vi "OAT Online Spectral Map with Resample.vi"(0 "scaled signal [EU]":waveform(dbl)={"t0"=timestamp(0 s since 1904-01-01), "dt"=0.0, "Y"=[]}, 1 "dB On (T)":bool=TRUE, 2 "reset? (True)":bool=TRUE, 5 "speed profile":T5 {"speed [RPM]" format="%.2f"; "time [s]" format="%.2f"}, 7 "pulse/revolution (1)":i32=1, 11 "error in (no error)":errorcluster, 12 "max order":i32, 13 "config":T1 {"range (auto)"."step" format="%.2f"; "range (auto)"."end" format="%.2f"; "range (auto)"."start" format="%.2f"}, 14 "window info":T2={"window type"=10, "window length"=2048} {"window type" items=["None"=0, "Hanning"=1, "Hamming"=2, "Blackman-Harris"=3, "Exact Blackman"=4, "Blackman"=5, "Flat Top"=6, "4 Term B-Harris"=7, "7 Term B-Harris"=8, "Low Sidelobe"=9, "Gaussian"=62]; "window length" min=0}) -> (4 "spectral map":dbl[][](array[numeric]) format="%.2f", 6 "scales":T4 {"Y scale"."multiplier" format="%.2f"; "Y scale"."offset" format="%.2f"; "X scale"."multiplier" format="%.2f"; "X scale"."offset" format="%.2f"}, 8 "unit labels":T3, 10 "finished":bool, 15 "error out":errorcluster)   [LabVIEW 2017]
doc: "Computes the <B>spectral map</B> of <B>scaled signal [EU]</B> based on the resampling method. This VI continuously computes <B>spectral map</B>."
uses:
  <vilib>/addons/Sound and Vibration/Order Analysis/Tach Process/SubVIs/speed profile.ctl
  <vilib>/addons/Sound and Vibration/Order Analysis/Ref Gabor Order Tracking/window information.ctl
  <vilib>/addons/Sound and Vibration/Order Analysis/Resample Order Tracking/OAT Convert to Even Angle Signal (1 Channel).vi
  <vilib>/Waveform/WDTOps.llb/WDT Waveform Duration DBL.vi
  <vilib>/addons/Sound and Vibration/Order Analysis/Resample Order Tracking/SoundVib_Resampling.lvlib
  <vilib>/addons/Sound and Vibration/Order Analysis/Resample Order Tracking/SoundVib_OrderTracking.lvlib
  <vilib>/addons/Sound and Vibration/Order Analysis/Gabor Order Tracking/SoundVib_Gabor.lvlib
  <vilib>/addons/Sound and Vibration/Order Analysis/Tach Process/SoundVib_TachProcess.lvlib
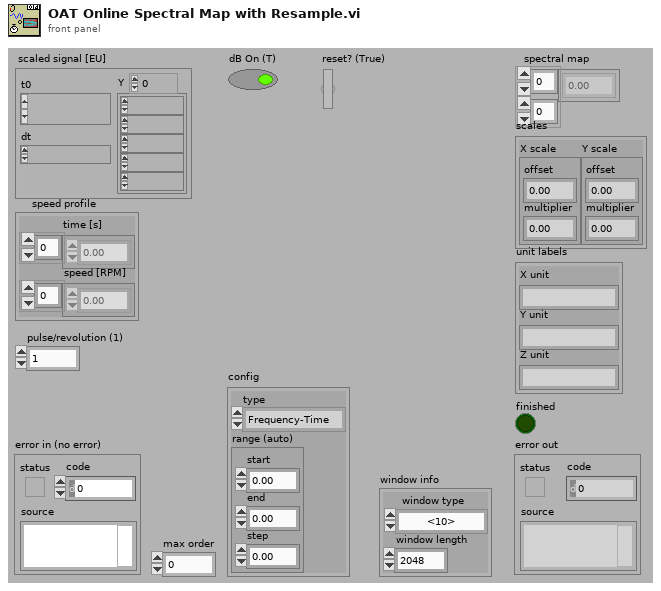
[diagram p1: front panel]
types:
  T1 = cluster{"type":enum16{"Frequency-Time", "Frequency-RPM", "Order-RPM"}, "range (auto)":cluster{"start":dbl, "end":dbl, "step":dbl}}
  T2 = typedef "SoundVib_Gabor.lvlib/window information.ctl" = cluster{"window type":u32, "window length":i32}
  T3 = cluster{"X unit":string, "Y unit":string, "Z unit":string}
  T4 = cluster{"X scale":cluster{"offset":dbl, "multiplier":dbl}, "Y scale":cluster{"offset":dbl, "multiplier":dbl}}
  T5 = typedef "SoundVib_TachProcess.lvlib/speed profile.ctl" = cluster{"time [s]":dbl[], "speed [RPM]":dbl[]}
  T6 = cluster{"Z axis unit label":string, "Z axis unit label":string, "Z axis unit label":string}
  T7 = cluster{"type":enum16{"Frequency-Time", "Frequency-RPM", "Order-RPM"}, "range":cluster{"start":dbl, "end":dbl, "step":dbl}}
  T8 = enum16{"Frequency-Time", "Frequency-RPM", "Order-RPM"}
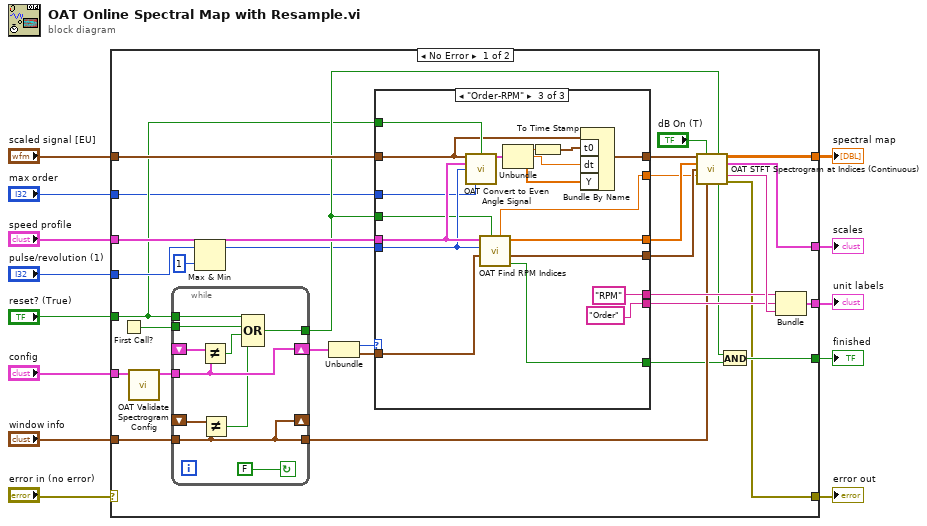
[diagram p0: block diagram]
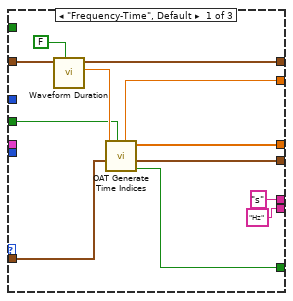
[diagram p2: hidden frame]
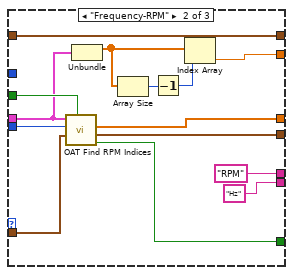
[diagram p3: hidden frame]
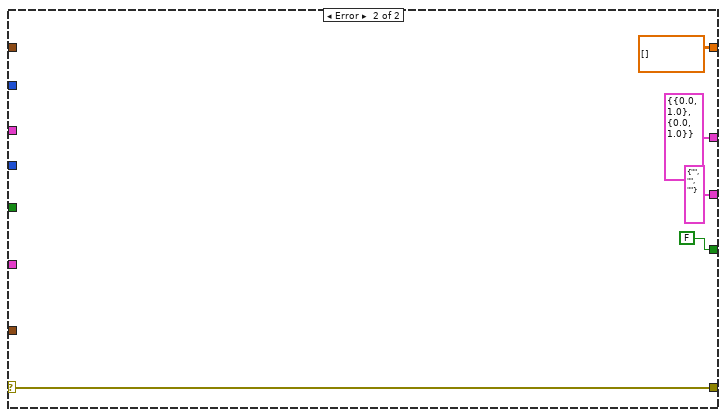
[diagram p4: hidden frame]
diagram:
  n1 = case shown="No Error" "error in (no error)" {
    selector: "error in (no error)" -> [_ w104]
    tunnel: "speed profile" -> [w44 _]
    tunnel: "scaled signal [EU]" -> [w43 _]
    tunnel: "pulse/revolution (1)" -> [w42 _]
    tunnel: [w36 dbl[][] [] ("spectral map")] -> w10
    tunnel: "window info" -> [w31 _]
    tunnel: [w27 FALSE] -> w8
    tunnel: [w26 T6 {"Z axis unit label"="", "Z axis unit label"="", "Z axis unit label"=""}] -> w7
    tunnel: "config" -> [w25 _]
    tunnel: "reset? (True)" -> [w23 _]
    tunnel: [w19 T4 {"X scale"={"offset"=0.0, "multiplier"=1.0}, "Y scale"={"offset"=0.0, "multiplier"=1.0}} ("scales")] -> w4
    tunnel: "max order" -> [w17 _]
    tunnel: [w16 w104] -> w1
    frame No Error {
      n2 = First Call?() -> (First Call?: T/F=w22:bool)
      n3 = call <vilib>:"OAT Validate Spectrogram Config.vi"("config"=w25) -> ("config"=w24:T7)  [unwired: 10 in]
      n4 = while {
        tunnel: w24 -> [w49]
        tunnel: w22 -> [w54]
        tunnel: w23 -> [w53]
        tunnel: [w51] -> w39
        shift-right: [w49] -> w37
        shift-left: _ -> [w48]
        shift-right: [w47] -> _
        shift-left: _ -> [w46]
        tunnel: w31 -> [w47]
        tunnel: [w47] -> w30
        stop <- FALSE continue-if-true
        n5 = Not Equal?(x=w48, y=w49) -> (x != y?=w52:bool)
        n6 = Not Equal?(x=w46, y=w47) -> (x != y?=w45:bool)
        n7 = Compound Arithmetic op=OR(w53, w54, w52, w45) -> (w51:bool)
      }
      n8 = Max & Min(x=w42, y=1) -> (max(x,y)=w15:i32)  [unwired: 1 out]
      n9 = Unbundle(w37) -> ("type"=w41:T8, "range"=w38:cluster{"start":dbl, "end":dbl, "step":dbl})
      n10 = case shown="\"Order-RPM\"" w41 {
        tunnel: w43 -> [w63 w78 w88]
        tunnel: [w62 w78 w83] -> w40
        tunnel: w44 -> [_ w71 w99]
        tunnel: w38 -> [w64 w80 w98]
        tunnel: w15 -> [_ w79 w97]
        tunnel: [w58 w77 w96] -> w21
        tunnel: w39 -> [w56 w76 w95]
        tunnel: [w59 w75 w94] -> w28
        tunnel: [w57 w74 w93] -> w20
        tunnel: ["s" ("Z axis unit label") "RPM" ("Z axis unit label") "RPM" ("Z axis unit label")] -> w33
        tunnel: ["Hz" ("Z axis unit label") "Hz" ("Z axis unit label") "Order" ("Z axis unit label")] -> w32
        tunnel: w17 -> [_ _ w82]
        tunnel: w23 -> [_ _ w90]
        tunnel: [w55 w67 w89] -> w18
        frame "Frequency-Time", Default {
          n11 = call-poly <vilib>:"Waveform Duration.vi"("open interval? (T)"=FALSE, "waveform in"=w63) -> ("duration"=w60:dbl, "waveform out"=w62:waveform(dbl))  [unwired: 7 in, 1 out]
          n12 = call <vilib>:"OAT Generate Time Indices.vi"("reset? (True)"=w56, "steps"=w64, "duration"=w60) -> ("finished"=w59:bool, "scale"=w57:cluster{"offset":dbl, "multiplier":dbl}, "time indices"=w58:dbl[], "signal processed"=w55:dbl)  [unwired: 5 in]
        }
        frame "Frequency-RPM" {
          n13 = call <vilib>:"OAT Find RPM Indices.vi"("reset? (True)"=w76, "RPM range"=w80, "pulse/revolution (1)"=w79, "speed profile"=w71) -> ("finished"=w75:bool, "RPM scale"=w74:cluster{"offset":dbl, "multiplier":dbl}, "time indices"=w77:dbl[])  [unwired: 3 in, 2 out]
          n14 = Unbundle(w71) -> ("time [s]"=w70:dbl[])  [unwired: 1 out]
          n15 = Array Size(array=w70) -> (size(s)=w69:i32)
          n16 = Decrement(x=w69) -> (x-1=w68:i32)
          n17 = Index Array(array=w70, index=w68) -> (element=w67:dbl)
        }
        frame "Order-RPM" {
          n18 = call-poly <vilib>:"OAT Convert to Even Angle Signal.vi"("scaled signal [EU]"=w88, "reset? (F)"=w90, "speed profile"=w99, "pulse/revolution (1)"=w97, "max order (auto)"=w82) -> ("even-angle signal"=w87:cluster{"r0":dbl, "dr":dbl, "Y":dbl[]})  [unwired: 6 in, 4 out]
          n19 = call <vilib>:"OAT Find RPM Indices.vi"("reset? (True)"=w95, "RPM range"=w98, "pulse/revolution (1)"=w97, "speed profile"=w99) -> ("finished"=w94:bool, "RPM scale"=w93:cluster{"offset":dbl, "multiplier":dbl}, "rev indices"=w96:dbl[], "last revolution"=w89:dbl)  [unwired: 3 in, 1 out]
          n20 = Unbundle(w87) -> ("r0"=w86:dbl, "dr"=w85:dbl, "Y"=w84:dbl[])
          n21 = To Time Stamp(1:w86) -> (0:w81:timestamp)
          n22 = Bundle By Name(cluster=w88, "t0"=w81, "dt"=w85, "Y"=w84) -> (w83:waveform(dbl))
        }
      }
      n23 = call <vilib>:"OAT STFT Spectrogram at Indices (Continuous).vi"("resampled signal"=w40, "dB On (T)"="dB On (T)", "reset? (True)"=w39, "time indices"=w21, "X scale in"=w20, "last indices"=w18, "spectral settings"=w30) -> ("spectral map"=w36:dbl[][], "scales"=w19:T4, "Z axis unit label"=w34:string, "finished"=w29:bool, "error out"=w16:errorcluster)  [unwired: 4 in]
      n24 = And(x=w29, y=w28) -> (x .and. y?=w27:bool)
      n25 = Bundle("Z axis unit label"=w33, "Z axis unit label"=w32, "Z axis unit label"=w34) -> (w26:T6)  [unwired: 1 in]
    }
    frame Error {
    }
  }
  "spectral map" <- w10
  "scales" <- w4
  "unit labels" <- w7
  "finished" <- w8
  "error out" <- w1
